vi "Write Cylinder.vi"(10 "ActuatorCylinder":refnum<class "IActuatorCylinder.lvclass">, 11 "FlowControlActuator in":refnum<class "FlowControlActuator.lvclass">) -> (3 "FlowControlActuator out":refnum<class "FlowControlActuator.lvclass">)   [LabVIEW 2015, in "FlowControlActuator.lvclass"]
uses:
  FlowControlActuator.lvclass
  ActuatorCylinder/IActuatorCylinder/IActuatorCylinder.lvclass
  FlowControlActuator.lvclass/FlowControlActuator.ctl
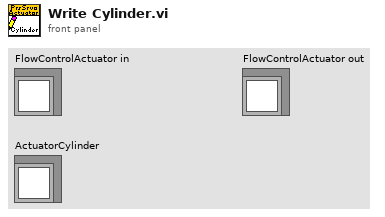
[diagram p1: front panel]
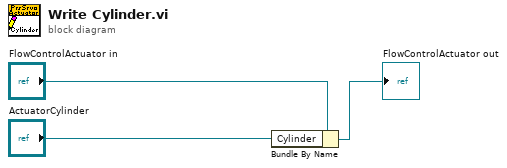
[diagram p0: block diagram]
diagram:
  n1 = Bundle By Name(cluster="FlowControlActuator in", "Cylinder"="ActuatorCylinder") -> (→"FlowControlActuator out":refnum<class "FlowControlActuator.lvclass">)
